vi "Is Class Dottable.vi"(9 "Parent Class Name":string, 10 "Property Name":string, 11 "ClassName":string) -> (1 "Not Found":bool, 2 "Not Dottable":bool, 3 "Dottable":bool)   [LabVIEW 2023]
doc: "In properties list, if a property returns a reference, this VI will tell you if the reference has a list of \"dottable\" properties to insert into the properties list.\n\nThis list was compiled manually for LV2019, and probably has errors and may be invalid for future versions of LV (which will hopefully return a complete list of properties when asked),"
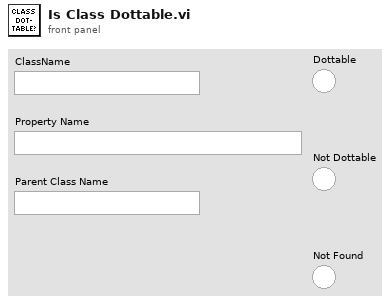
[diagram p1: front panel]
types:
  T1 = cluster{"Undotted Property":string, "Bare Property":string, "Is dotted?":bool, "Dot depth":i32, "Indent":i32, "Property Hierarchy":string[], "Parents":string[]}
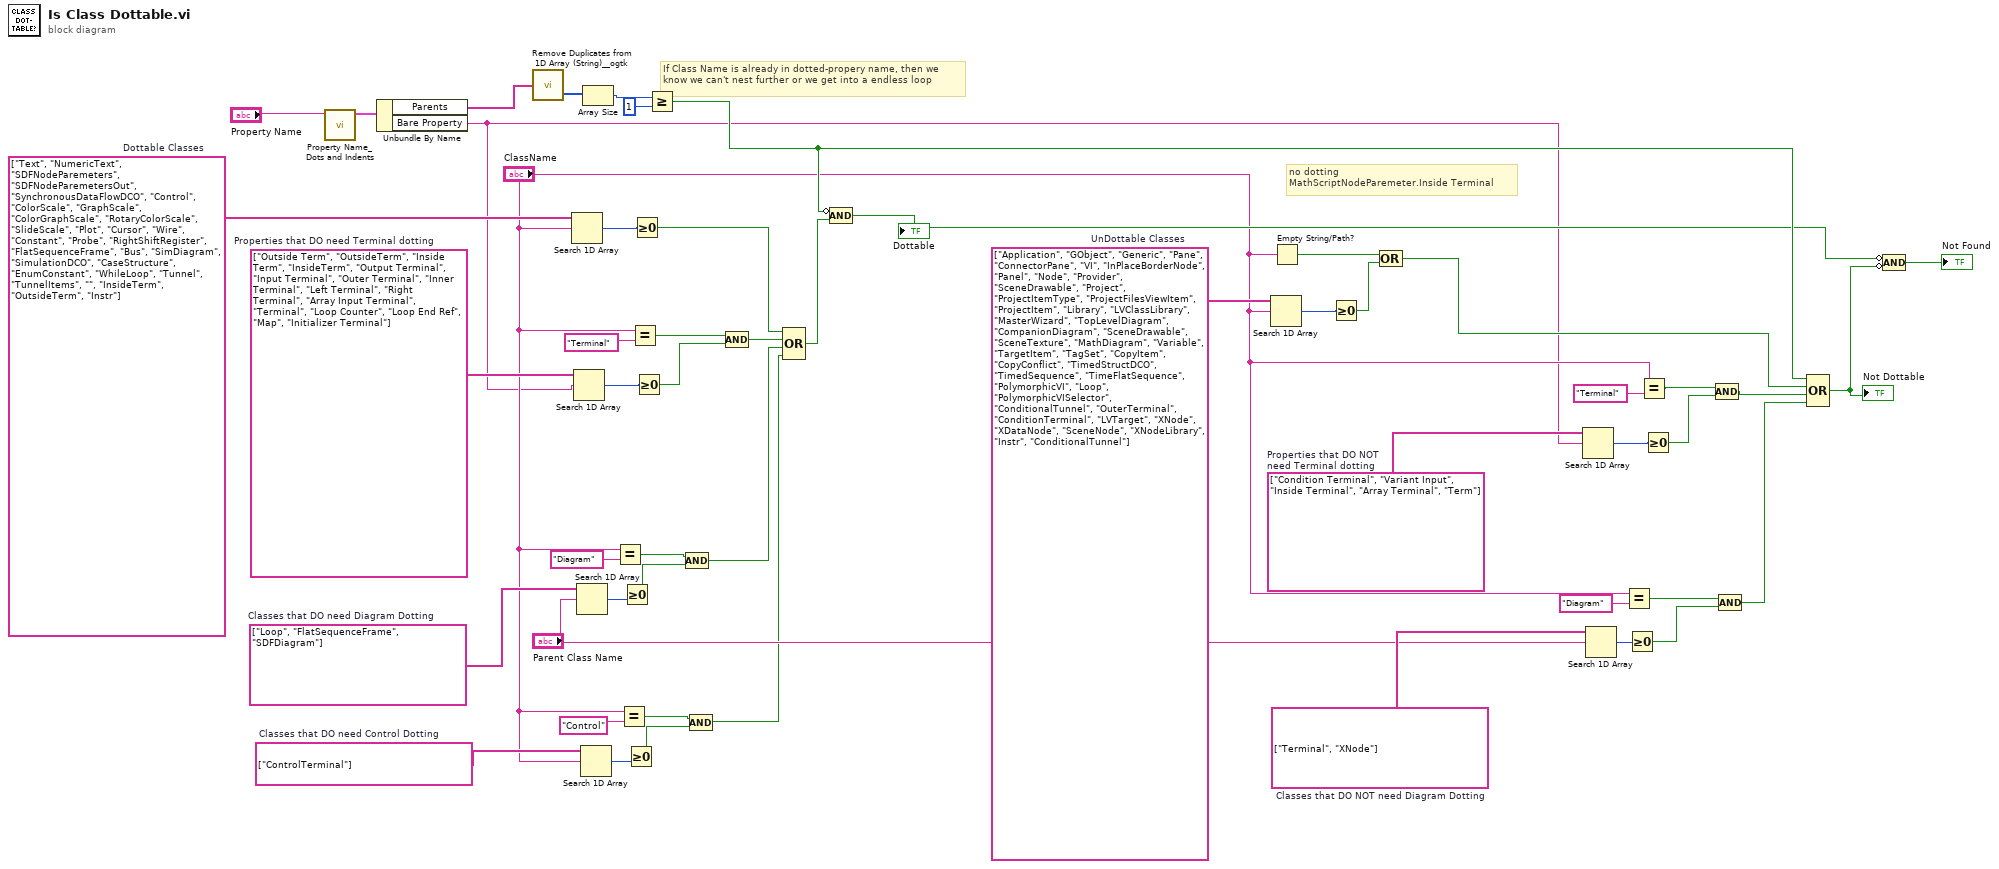
[diagram p0: block diagram]
diagram:
  w6 = string[] ["ControlTerminal"]  # Classes that DO need Control Dotting
  w26 = string[] ["Condition Terminal", "Variant Input", "Inside Terminal", "Array Terminal", "Term"]  # Properties that DO NOT need Terminal dotting
  w27 = string[] ["Terminal", "XNode"]  # Classes that DO NOT need Diagram Dotting
  w44 = string[] ["Outside Term", "OutsideTerm", "Inside Term", "InsideTerm", "Output Terminal", "Input Terminal", "Outer Terminal", "Inner Terminal", "Left Terminal", "Right Terminal", "Array Input Terminal", "Terminal", "Loop Counter", "Loop End Ref", "Map", "Initializer Terminal"]  # Properties that DO need Terminal dotting
  w39 = string[] ["Loop", "FlatSequenceFrame", "SDFDiagram"]  # Classes that DO need Diagram Dotting
  w49 = string[] ["Application", "GObject", "Generic", "Pane", "ConnectorPane", "VI", "InPlaceBorderNode", "Panel", "Node", "Provider", "SceneDrawable", "Project", "ProjectItemType", "ProjectFilesViewItem", "ProjectItem", "Library", "LVClassLibrary", "MasterWizard", "TopLevelDiagram", "CompanionDiagram", "SceneDrawable", "SceneTexture", "MathDiagram", "Variable", "TargetItem", "TagSet", "CopyItem", "CopyConflict", "TimedStructDCO", "TimedSequence", "TimeFlatSequence", "PolymorphicVI", "Loop", "PolymorphicVISelector", "ConditionalTunnel", "OuterTerminal", "ConditionTerminal", "LVTarget", "XNode", "XDataNode", "SceneNode", "XNodeLibrary", "Instr", "ConditionalTunnel"]  # UnDottable Classes
  w52 = string[] ["Text", "NumericText", "SDFNodeParemeters", "SDFNodeParemetersOut", "SynchronousDataFlowDCO", "Control", "ColorScale", "GraphScale", "ColorGraphScale", "RotaryColorScale", "SlideScale", "Plot", "Cursor", "Wire", "Constant", "Probe", "RightShiftRegister", "FlatSequenceFrame", "Bus", "SimDiagram", "SimulationDCO", "CaseStructure", "EnumConstant", "WhileLoop", "Tunnel", "TunnelItems", "", "InsideTerm", "OutsideTerm", "Instr"]  # Dottable Classes
  # "If Class Name is already in dotted-propery name, then we know we can't nest further or we get into a endless loop"
  # "no dotting\nMathScriptNodeParemeter.Inside Terminal"
  n1 = call "Property Name_Dots and Indents.vi"("Property"="Property Name") -> ("Cluster"=w3:T1)  [unwired: 10 in]
  n2 = Unbundle By Name(w3) -> ("Parents"=w1:string[], "Bare Property"=w2:string)
  n3 = call <userlib>:"Remove Duplicates from 1D Array (String)__ogtk.vi"("Input Array"=w1) -> ("indices of removed elements"=w16:i32[])  [unwired: 1 out]
  n4 = Search 1D Array(1D array=w52, element="ClassName") -> (index of element=w51:i32)  [unwired: 1 in]
  n5 = Search 1D Array(1D array=w44, element=w2) -> (index of element=w45:i32)  [unwired: 1 in]
  n6 = Search 1D Array(1D array=w39, element="Parent Class Name") -> (index of element=w38:i32)  [unwired: 1 in]
  n7 = Search 1D Array(1D array=w6, element="ClassName") -> (index of element=w7:i32)  [unwired: 1 in]
  n8 = Array Size(array=w16) -> (size(s)=w15:i32)
  n9 = Equal?(x="ClassName", y="Diagram") -> (x = y?=w35:bool)
  n10 = Equal?(x="ClassName", y="Control") -> (x = y?=w9:bool)
  n11 = Greater Or Equal To 0?(x=w38) -> (x >= 0?=w34:bool)
  n12 = Greater Or Equal To 0?(x=w7) -> (x >= 0?=w10:bool)
  n13 = Equal?(x="ClassName", y="Terminal") -> (x = y?=w42:bool)
  n14 = Greater Or Equal To 0?(x=w51) -> (x >= 0?=w40:bool)
  n15 = Greater Or Equal To 0?(x=w45) -> (x >= 0?=w37:bool)
  n16 = Greater Or Equal?(x=w15, y=1) -> (x >= y?=w12:bool)
  n17 = Compound Arithmetic op=AND(w35, w34) -> (w33:bool)
  n18 = Compound Arithmetic op=AND(w9, w10) -> (w4:bool)
  n19 = Compound Arithmetic op=AND(w42, w37) -> (w41:bool)
  n20 = Compound Arithmetic op=OR(w40, w41, w33, w4) -> (w13:bool)
  n21 = Compound Arithmetic op=AND(invert w12, w13) -> (w11:bool)
  "Dottable" <- w11
  n22 = Search 1D Array(1D array=w49, element="ClassName") -> (index of element=w50:i32)  [unwired: 1 in]
  n23 = Empty String/Path?(string/path="ClassName") -> (empty?=w47:bool)
  n24 = Greater Or Equal To 0?(x=w50) -> (x >= 0?=w46:bool)
  n25 = Compound Arithmetic op=OR(w47, w46) -> (w19:bool)
  n26 = Search 1D Array(1D array=w26, element=w2) -> (index of element=w25:i32)  [unwired: 1 in]
  n27 = Search 1D Array(1D array=w27, element="Parent Class Name") -> (index of element=w28:i32)  [unwired: 1 in]
  n28 = Equal?(x="ClassName", y="Diagram") -> (x = y?=w31:bool)
  n29 = Greater Or Equal To 0?(x=w28) -> (x >= 0?=w32:bool)
  n30 = Equal?(x="ClassName", y="Terminal") -> (x = y?=w22:bool)
  n31 = Greater Or Equal To 0?(x=w25) -> (x >= 0?=w29:bool)
  n32 = Compound Arithmetic op=AND(w22, w29) -> (w21:bool)
  n33 = Compound Arithmetic op=AND(w31, w32) -> (w20:bool)
  n34 = Compound Arithmetic op=OR(w12, w19, w21, w20) -> (w18:bool)
  "Not Dottable" <- w18
  n35 = Compound Arithmetic op=AND(invert w11, invert w18) -> (→"Not Found":bool)
